vi "Read Values DVR.vi"(8 "error in (no error)":errorcluster, 11 "DAQmx-Bus_DBLType in":refnum<class "DAQmx-Bus_Bool_Type.lvclass">) -> (0 "error out":errorcluster, 2 "Values DVR":refnum<data-value>, 3 "DAQmx-Bus_DBLType out":refnum<class "DAQmx-Bus_Bool_Type.lvclass">)   [LabVIEW 2021, in "DAQmx-Bus_Bool_Type.lvclass"]
uses:
  DAQmx-Bus_Bool_Type.lvclass
  DAQmx-Bus_Bool_Type.lvclass/DAQmx-Bus_Bool_Type.ctl
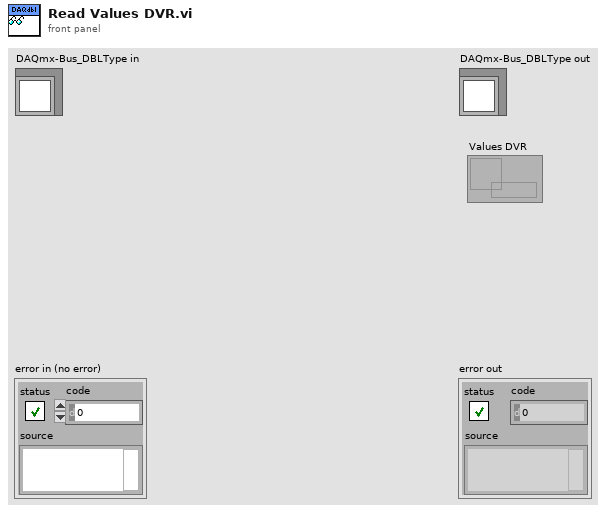
[diagram p1: front panel]
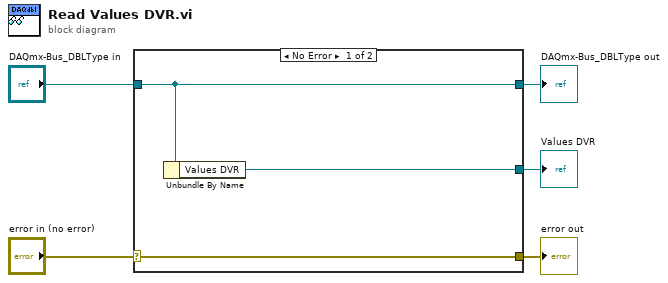
[diagram p0: block diagram]
diagram:
  n1 = case shown="No Error" "error in (no error)" {
    selector: "error in (no error)" -> [w8 w9]
    tunnel: [w8 w9] -> w4
    tunnel: [w7 w10] -> w2
    tunnel: "DAQmx-Bus_DBLType in" -> [w7 w10]
    tunnel: [w6 _] -> w1
    frame No Error {
      n2 = Unbundle By Name(w7) -> ("Values DVR"=w6:refnum<data-value>)
    }
    frame Error {
    }
  }
  "error out" <- w4
  "DAQmx-Bus_DBLType out" <- w2
  "Values DVR" <- w1
